vi "Printing - Custom Device Async Loop Stopped.vi"(8 "error in (no error)":errorcluster, 11 "Name":string) -> (0 "error out":errorcluster)   [LabVIEW 2015, in "Shared Variable Custom Device.lvlib"]
uses:
  Shared Variable Custom Device.lvlib
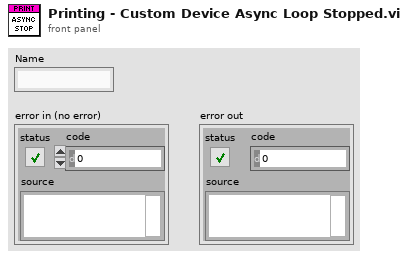
[diagram p1: front panel]
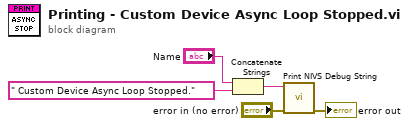
[diagram p0: block diagram]
diagram:
  n1 = Concatenate Strings("Name", " Custom Device Async Loop Stopped." ("string")) -> (w4:string)
  n2 = call "Print NIVS Debug String.vi"("error in (no error)"="error in (no error)", "Debug String"=w4) -> ("error out"=→"error out":errorcluster)  [unwired: 8 in]
